vi "wd_addRecordInOneNode (DBL).vi"(6 "length":u64, 7 "data":dbl[](array[numeric]), 8 "error in (no error)":errorcluster, 9 "start":u64, 10 "datalog postion":i64, 11 "meta in":T1={"TargetFile"=path "", "StreamMode"=enum."File", "Append?"=FALSE, "ChunkSize"=0, "TimeColumnMode"=enum."Empty", "TimestampFormat"="", "AbsoluteTime?"=FALSE, "FileAttribute "={"Creator"="", "Title"="", "SheetName"=""}, "Column"=[], "FileRef"=refnum, "MemoryRef"=[], "RecordInfo"=[], " ChannelPreviousInfo"=[], "ChannelFirstRecord"=[], "PredefinedFormattedValueLength"=20, "DiskTemplate"={"XMLRef"=[refnum, refnum, refnum, refnum, refnum, refnum], "ZipPath"=path "", "MetaFile"={"Ref"=refnum, "NextRow"=0, "NextPosition"=0, "Block"=[]}, "TempFolder"=path ""}}) -> (0 "error out":errorcluster, 3 "meta out":T1={"TargetFile"=path "", "StreamMode"=enum."File", "Append?"=FALSE, "ChunkSize"=0, "TimeColumnMode"=enum."Empty", "TimestampFormat"="", "AbsoluteTime?"=FALSE, "FileAttribute "={"Creator"="", "Title"="", "SheetName"=""}, "Column"=[], "FileRef"=refnum, "MemoryRef"=[], "RecordInfo"=[], " ChannelPreviousInfo"=[], "ChannelFirstRecord"=[], "PredefinedFormattedValueLength"=20, "DiskTemplate"={"XMLRef"=[refnum, refnum, refnum, refnum, refnum, refnum], "ZipPath"=path "", "MetaFile"={"Ref"=refnum, "NextRow"=0, "NextPosition"=0, "Block"=[]}, "TempFolder"=path ""}}, 4 "data subset":dbl[](array[numeric]))   [LabVIEW 2017, in "NI_ExcelFile.lvlib"]
uses:
  <vilib>/express/express shared/NI_ExcelFile/NI_ExcelFile.lvlib
  <vilib>/express/express shared/NI_ExcelFile/Ctrls/MainData.ctl
  <vilib>/express/express shared/NI_ExcelFile/Ctrls/StreamMode.ctl
  <vilib>/express/express shared/NI_ExcelFile/Ctrls/TimeColumnMode.ctl
  <vilib>/express/express shared/NI_ExcelFile/Ctrls/FileAttribute.ctl
  <vilib>/express/express shared/NI_ExcelFile/Ctrls/Columns.ctl
  <vilib>/express/express shared/NI_ExcelFile/Ctrls/ColumnInfo.ctl
  <vilib>/express/express shared/NI_ExcelFile/Ctrls/DataType.ctl
  <vilib>/express/express shared/NI_ExcelFile/Ctrls/wd_recordInfo.ctl
  <vilib>/express/express shared/NI_ExcelFile/Ctrls/disk_TemplateFile.ctl
  <vilib>/express/express shared/NI_ExcelFile/Ctrls/meta_file.ctl
  <vilib>/express/express shared/NI_ExcelFile/Ctrls/meta_Block.ctl
  <vilib>/express/express shared/NI_ExcelFile/Ctrls/meta_BlockType.ctl
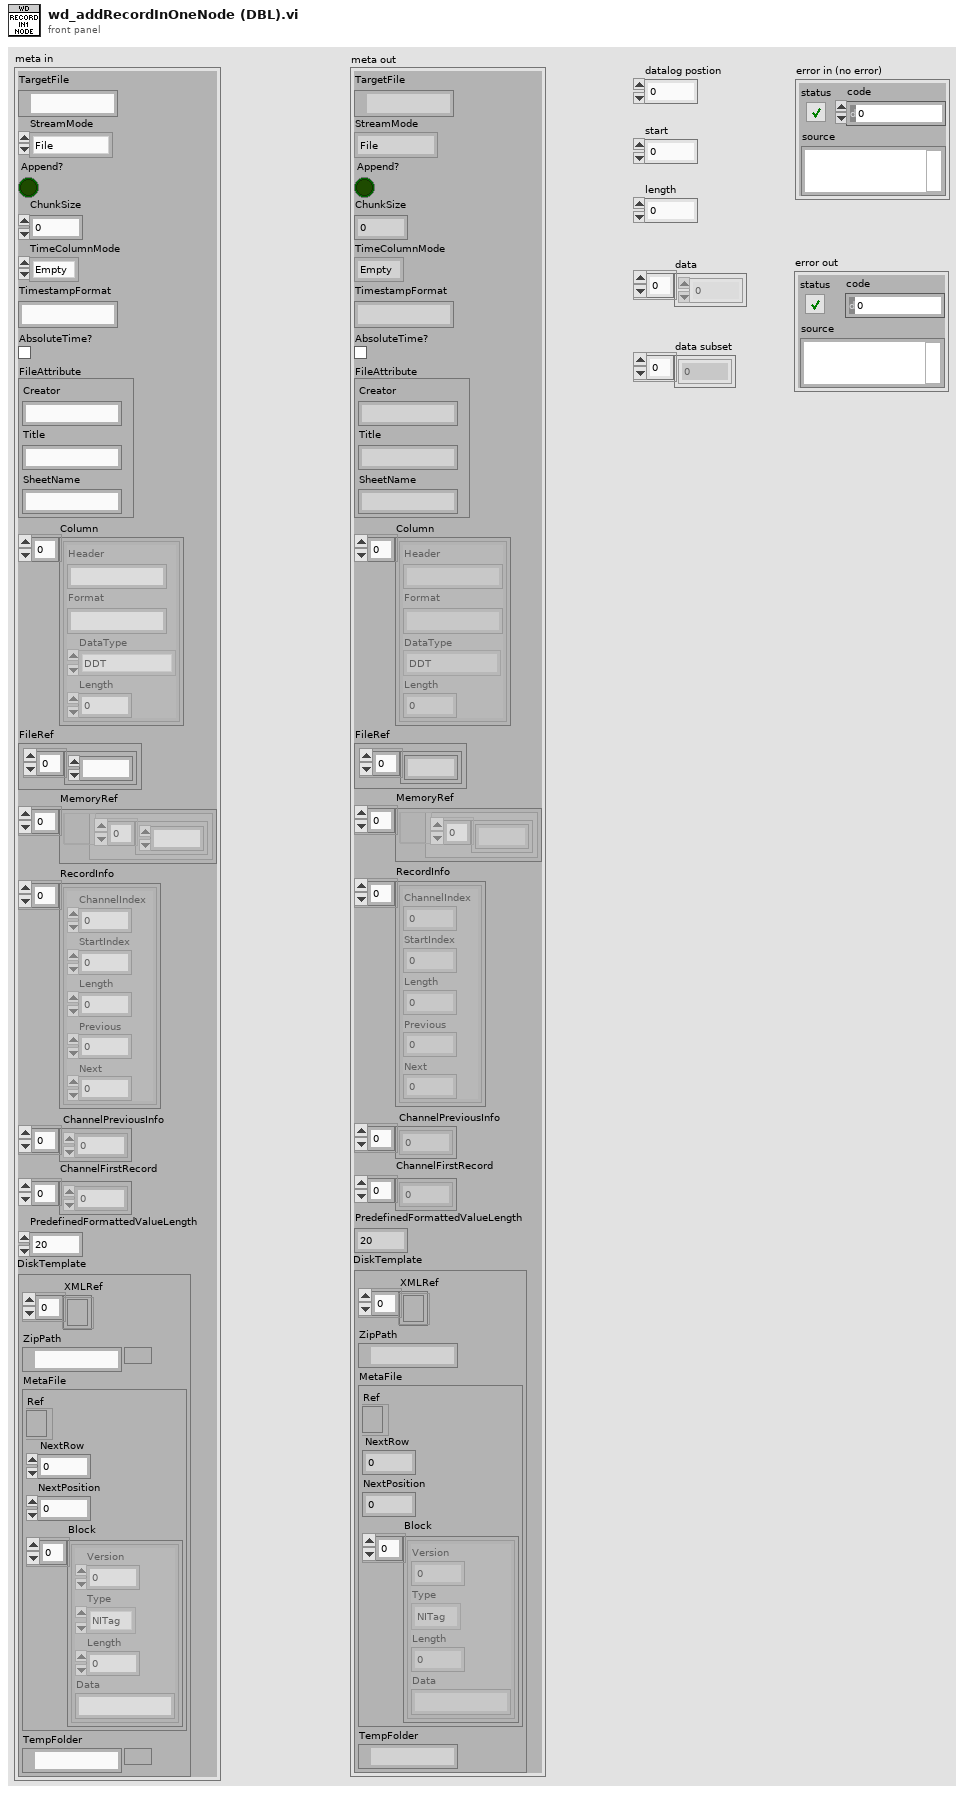
[diagram p1: front panel]
types:
  T1 = typedef "NI_ExcelFile.lvlib/MainData.ctl" = cluster{"TargetFile":path, "StreamMode":T2, "Append?":bool, "ChunkSize":u64, "TimeColumnMode":T3, "TimestampFormat":string, "AbsoluteTime?":bool, "FileAttribute ":T4, "Column":T5, "FileRef":refnum<k1>, "MemoryRef":refnum<data-value>[], "RecordInfo":T8[], " ChannelPreviousInfo":u32[], "ChannelFirstRecord":u32[], "PredefinedFormattedValueLength":i64, "DiskTemplate":T9}
  T2 = typedef "NI_ExcelFile.lvlib/StreamMode.ctl" = enum16{"File", "Memory"}
  T3 = typedef "NI_ExcelFile.lvlib/TimeColumnMode.ctl" = enum16{"Empty", "OnePerCh", "One"}
  T4 = typedef "NI_ExcelFile.lvlib/FileAttribute.ctl" = cluster{"Creator":string, "Title":string, "SheetName":string}
  T5 = typedef "NI_ExcelFile.lvlib/Columns.ctl" = T6[]
  T6 = typedef "NI_ExcelFile.lvlib/ColumnInfo.ctl" = cluster{"Header":string, "Format":string, "DataType":T7, "Length":u64}
  T7 = typedef "NI_ExcelFile.lvlib/DataType.ctl" = enum16{"DDT", "WFM", "Array of STR", "Array of DBL", "Array of I8", "Array of I16", "Array of I32", "Array of I64", "Array of SGL", "Array of U8", "Array of U16", "Array of U32", "Array of U64", "Array of Time"}
  T8 = typedef "NI_ExcelFile.lvlib/wd_recordInfo.ctl" = cluster{"ChannelIndex":u32, "StartIndex":u64, "Length":u64, "Previous":i32, "Next":i32}
  T9 = typedef "NI_ExcelFile.lvlib/disk_TemplateFile.ctl" = cluster{"XMLRef":refnum<file>[], "ZipPath":path, "MetaFile":T10, "TempFolder":path}
  T10 = typedef "NI_ExcelFile.lvlib/meta_file.ctl" = cluster{"Ref":refnum<file>, "NextRow":i32, "NextPosition":i64, "Block":T11[]}
  T11 = typedef "NI_ExcelFile.lvlib/meta_Block.ctl" = cluster{"Version":u16, "Type":T12, "Length":i32, "Data":string}
  T12 = typedef "NI_ExcelFile.lvlib/meta_BlockType.ctl" = enum16{"NITag", "File", "Column"}
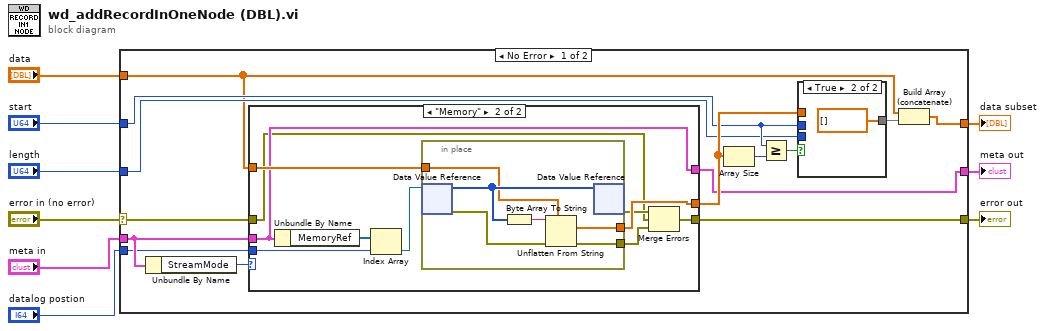
[diagram p0: block diagram]
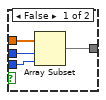
[diagram p2: hidden frame]
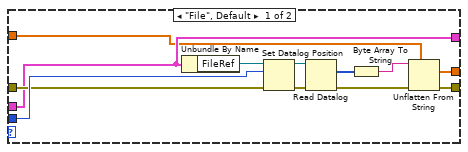
[diagram p3: hidden frame]
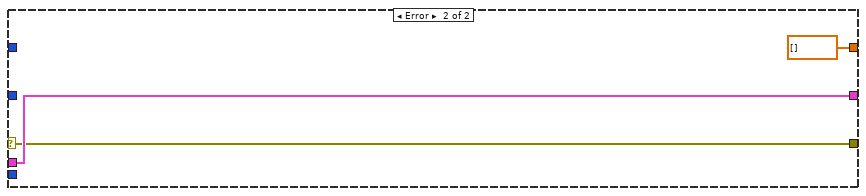
[diagram p4: hidden frame]
diagram:
  n1 = case shown="No Error" "error in (no error)" {
    selector: "error in (no error)" -> [w19 w58]
    tunnel: "datalog postion" -> [w18 _]
    tunnel: [w10 dbl[] [] ("data")] -> w8
    tunnel: "meta in" -> [w20 w59]
    tunnel: [w14 w59] -> w6
    tunnel: [w11 w58] -> w5
    tunnel: "data" -> [w13 _]
    tunnel: "start" -> [w16 _]
    tunnel: "length" -> [w15 _]
    frame No Error {
      n2 = Unbundle By Name(w20) -> ("StreamMode"=w23:T2)
      n3 = case shown="\"Memory\"" w23 {
        tunnel: w20 -> [w32 w46]
        tunnel: w19 -> [w34 w43]
        tunnel: w18 -> [w36 w47]
        tunnel: [w32 w46] -> w14
        tunnel: w13 -> [w31 w49]
        tunnel: [w30 w45] -> w17
        tunnel: [w29 w41] -> w11
        frame "File", Default {
          n4 = Unbundle By Name(w32) -> ("FileRef"=w35:refnum<k1>)
          n5 = Set Datalog Position(4:w34, 6:w36, 7:w35) -> (0:w40:errorcluster, 3:w37:refnum<k1>)  [unwired: 1 in]
          n6 = Read Datalog(4:w40, 7:w37) -> (0:w33:errorcluster, 2:w38:u8[])  [unwired: 1 in, 1 out]
          n7 = Byte Array To String(unsigned byte array=w38) -> (string=w39:string)
          n8 = Unflatten From String(type=w31, binary string=w39, error in (no error)=w33) -> (value=w30:dbl[], error out=w29:errorcluster)  [unwired: 2 in, 1 out]
        }
        frame "Memory" {
          n9 = Unbundle By Name(w46) -> ("MemoryRef"=w48:refnum<data-value>[])
          n10 = Index Array(array=w48, index=w47) -> (element=w50:refnum<data-value>)
          n11 = in-place {
            in-place-border: w49 -> [w53]
            in-place-border: [w52] -> w45
            in-place-border: [w51] -> w42
            n12 = in-place-dvr #1(w50) -> (w55:u8[], w54:errorcluster)
            n13 = Byte Array To String(unsigned byte array=w55) -> (string=w56:string)
            n14 = Unflatten From String(type=w53, binary string=w56, error in (no error)=w54) -> (value=w52:dbl[], error out=w51:errorcluster)  [unwired: 2 in, 1 out]
            n15 = in-place-dvr #1(w55) -> (w44:errorcluster)  [unwired: 1 out]
          }
          n16 = Merge Errors(w44, w43, w42) -> (w41:errorcluster)
        }
      }
      n17 = Array Size(array=w17) -> (size(s)=w22:i32)
      n18 = Greater Or Equal?(x=w16, y=w22) -> (x >= y?=w21:bool)
      n19 = case shown="True" w21 {
        tunnel: w17 -> [w27 _]
        tunnel: w16 -> [w26 _]
        tunnel: w15 -> [w25 _]
        tunnel: [w24 dbl[] []] -> w12
        frame False {
          n20 = Array Subset(array=w27, index=w26, length=w25) -> (w24:dbl[])
        }
        frame True {
        }
      }
      n21 = Build Array (concatenate)(w13, w12) -> (w10:dbl[])
    }
    frame Error {
    }
  }
  "data subset" <- w8
  "meta out" <- w6
  "error out" <- w5
